vi "Configure Range Table (Harmonic).vi"(0 "VISA resource name":refnum<visa-resource-name>, 1 "Enable Tone Measurement":bool[](array[boolean])=[TRUE, TRUE, TRUE, TRUE, TRUE, TRUE, TRUE, TRUE, TRUE, TRUE], 2 "Frequency List":dbl[](array[numeric])=[1000000000.0, 1000000000.0, 1000000000.0, 1000000000.0, 1000000000.0, 1000000000.0, 1000000000.0, 1000000000.0, 1000000000.0, 1000000000.0], 3 "Manual Bandwidth (1E+6Hz)":dbl=1000000.0, 5 "Enable Range Table (F: Disable)":bool, 7 "Tone Number (1)":i32(ring)=1 items=["1"=1, "2"=2, "3"=3, "4"=4, "5"=5, "6"=6, "7"=7, "8"=8, "9"=9, "10"=10], 9 "Auto Bandwidth (T: Enable)":bool=TRUE, 11 "error in (no error)":errorcluster, 12 "Auto Dwell Time":bool[](array[boolean])=[FALSE, FALSE, TRUE, TRUE, TRUE, TRUE, TRUE, TRUE, TRUE, TRUE], 13 "Manual Dwell Time":dbl[](array[numeric])=[1.0, 1.0, 1.0, 1.0, 1.0, 1.0, 1.0, 1.0, 1.0, 1.0]) -> (4 "VISA resource name out":refnum<visa-resource-name>, 15 "error out":errorcluster)   [LabVIEW 2014, in "Agilent MXA Series.lvlib"]
doc: "Configures the range table for harmonic measurement type."
uses:
  Agilent MXA Series.lvlib
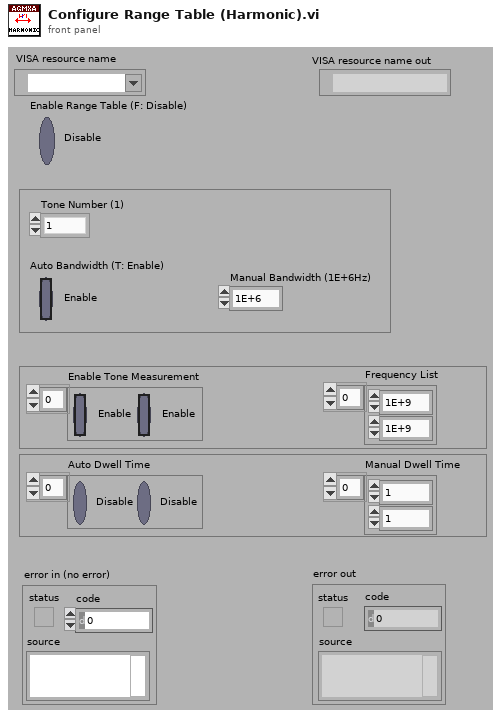
[diagram p1: front panel]
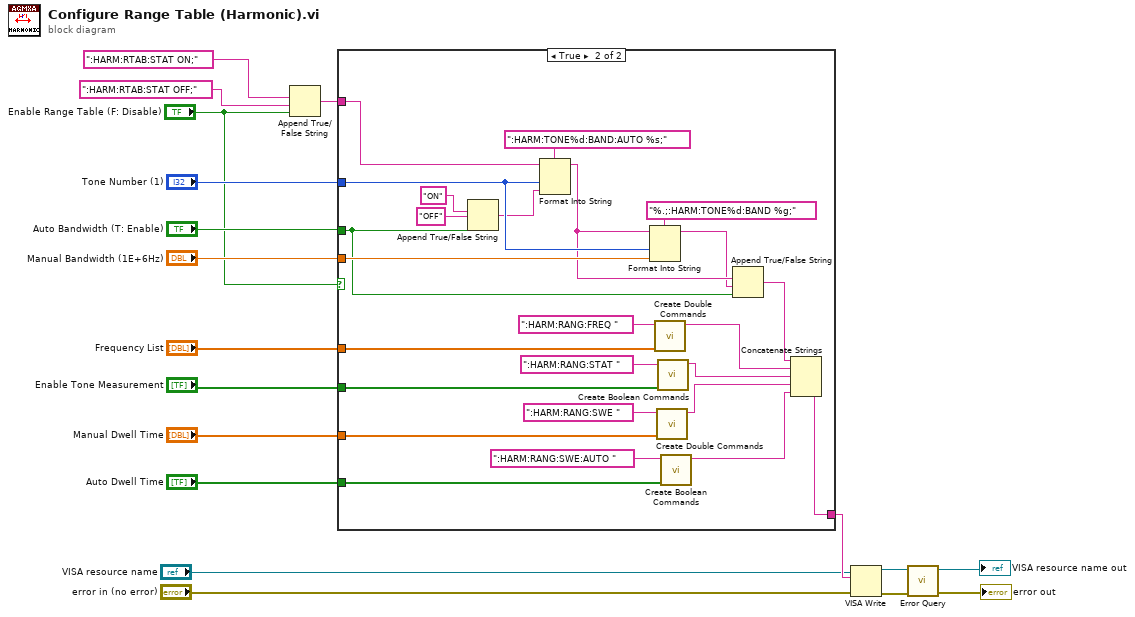
[diagram p0: block diagram]
diagram:
  n1 = Append True/False String(1:"Enable Range Table (F: Disable)", 2:":HARM:RTAB:STAT OFF;" ("true string"), 3:":HARM:RTAB:STAT ON;" ("true string")) -> (0:w2:string)  [unwired: 1 in]
  n2 = case shown="True" "Enable Range Table (F: Disable)" {
    tunnel: "Manual Dwell Time" -> [_ w44]
    tunnel: "Auto Dwell Time" -> [_ w42]
    tunnel: [w19 w20] -> w16
    tunnel: "Enable Tone Measurement" -> [_ w39]
    tunnel: "Frequency List" -> [_ w38]
    tunnel: "Tone Number (1)" -> [_ w34]
    tunnel: "Manual Bandwidth (1E+6Hz)" -> [_ w30]
    tunnel: "Auto Bandwidth (T: Enable)" -> [_ w29]
    tunnel: w2 -> [w19 w26]
    frame False {
    }
    frame True {
      n3 = Append True/False String(1:w29, 2:"OFF" ("true string"), 3:"ON" ("true string")) -> (0:w31:string)  [unwired: 1 in]
      n4 = Format Into String(format string=":HARM:TONE%d:BAND:AUTO %s;", initial string=w26, w34, w31) -> (resulting string=w28:string)  [unwired: 1 in, 1 out]
      n5 = Format Into String(format string="%.;:HARM:TONE%d:BAND %g;", initial string=w28, w34, w30) -> (resulting string=w27:string)  [unwired: 1 in, 1 out]
      n6 = call "Create Double Commands.vi"("Double Values"=w38, "Commands"=":HARM:RANG:FREQ ") -> ("Result"=w24:string)  [unwired: 9 in]
      n7 = call "Create Double Commands.vi"("Double Values"=w44, "Commands"=":HARM:RANG:SWE ") -> ("Result"=w22:string)  [unwired: 9 in]
      n8 = call "Create Boolean Commands.vi"("Boolean States"=w39, "Command"=":HARM:RANG:STAT " ("Commands")) -> ("Result String"=w23:string)  [unwired: 9 in]
      n9 = call "Create Boolean Commands.vi"("Boolean States"=w42, "Command"=":HARM:RANG:SWE:AUTO ") -> ("Result String"=w21:string)  [unwired: 9 in]
      n10 = Append True/False String(1:w29, 2:w27, 3:w28) -> (0:w25:string)  [unwired: 1 in]
      n11 = Concatenate Strings(w25, w24, w23, w22, w21) -> (w20:string)
    }
  }
  n12 = VISA Write(VISA resource name="VISA resource name", write buffer=w16, error in (no error)="error in (no error)") -> (VISA resource name out=w12:refnum<visa-resource-name>, error out=w13:errorcluster)  [unwired: 1 out]
  n13 = call "Error Query.vi"("error in (no error)"=w13, "VISA resource name"=w12) -> ("error out"=→"error out":errorcluster, "VISA resource name out"=→"VISA resource name out":refnum<visa-resource-name>)  [unwired: 6 in, 2 out]
